vi "Boiler.vi"() -> ()   [LabVIEW 2013]
doc: "This VI is a simulation of boiler controller.\nThere are the following states-\n-Initialize\n-Reset Lockout\n-Pre-purge\n-Pre-purge continued\n-Ignition\n-Prove the pilot\n-Start and Run\n-Start and Run contiuued\n-Shutdown and purge: After elapsed time of the state VI will again go back to the initialize state.\n-Stop: On pressing Stop the VI will stop working and all the controlls and indicator will go to default value.\n\nThis VI allow the user to start and stop the boiller.\nThe status is a event string.\nTime Count- count the time till the time elapsed."
uses:
  Controls/Boiler Controls.ctl
  Controls/Boiler Simulation Controls.ctl
  Controls/Boiler Status Indicators.ctl
  CarWash/USB Template (LV 8.6)/Car Wash/Controls/States.ctl
panel:
  in  "Stop":bool
  out "Boiler Status Indicators":T1 {"Time Count" format="%.2g"}
  in  "Boiler Simulation Controls":T2 {"Flame Sensor Value (%)" min=0.0 max=100.0 scale=0.0..100.0}
  in  "Boiler Controls":T3 {"Fuel Valve Position" min=0.0 max=100.0 scale=0.0..100.0 scale format="%.2f"}
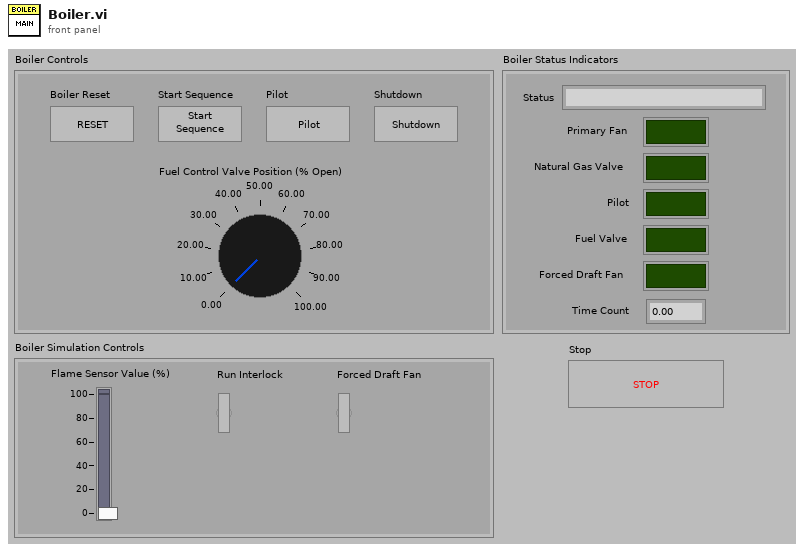
[diagram p1: front panel]
types:
  T1 = typedef "Boiler Status Indicators.ctl" = cluster{"Status":string, "Primary Fan":bool, "Natural Gas Valve":bool, "Pilot":bool, "Fuel Valve":bool, "Forced Draft Fan":bool, "Time Count":dbl}
  T2 = typedef "Boiler Simulation Controls.ctl" = cluster{"Flame Sensor Value (%)":dbl, "Run Interlock":bool, "Forced Draft Fan":bool}
  T3 = typedef "Boiler Controls.ctl" = cluster{"Boiler Reset":bool, "Start Sequence":bool, "Pilot":bool, "Shutdown":bool, "Fuel Valve Position":dbl}
  T4 = typedef "States.ctl" = enum16{"Initialize", "Start", "Reset Lockout", "Pre-Purge", "Pre-Perge Cont.", "Ignition", "Prove the Pilot", "Start and Run", "Run Cont.", "Shutdown and purge", "Purge", "Stop"}
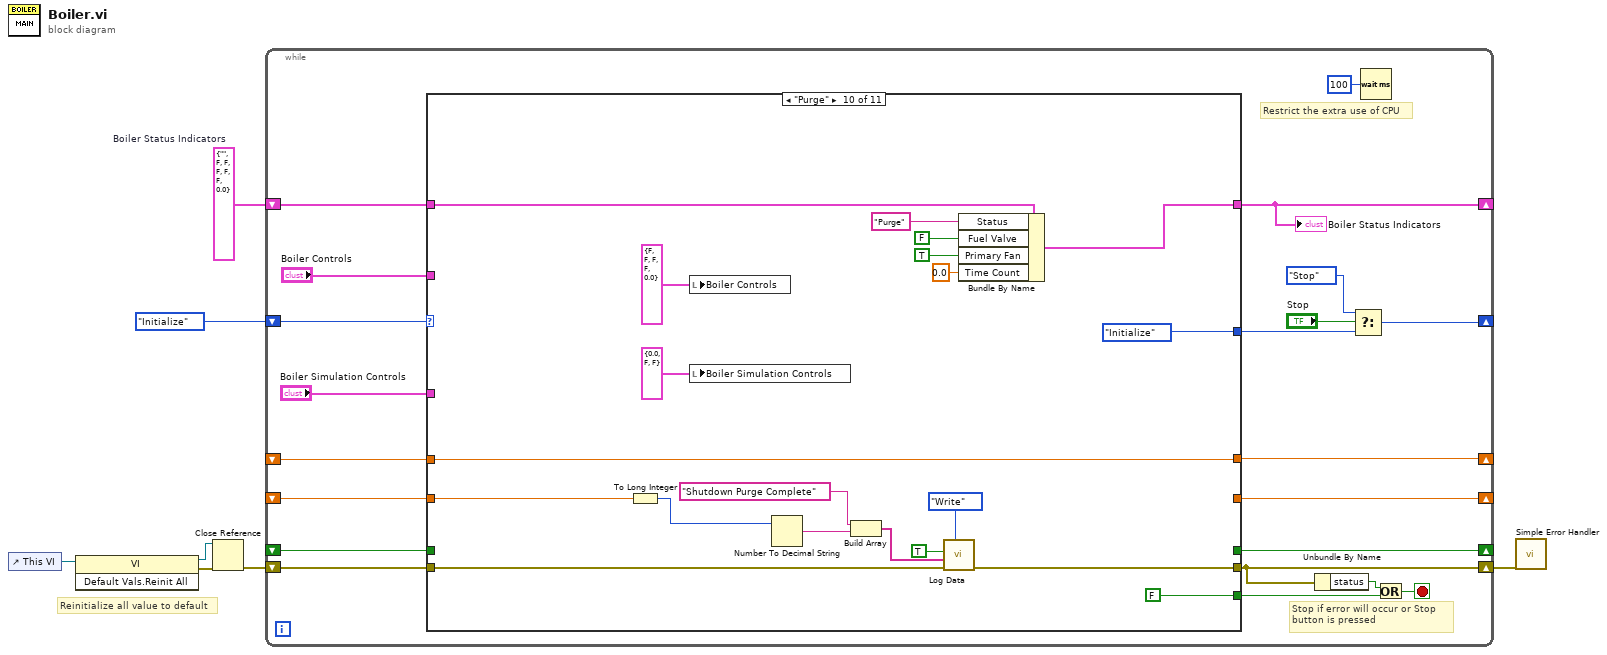
[diagram p0: block diagram]
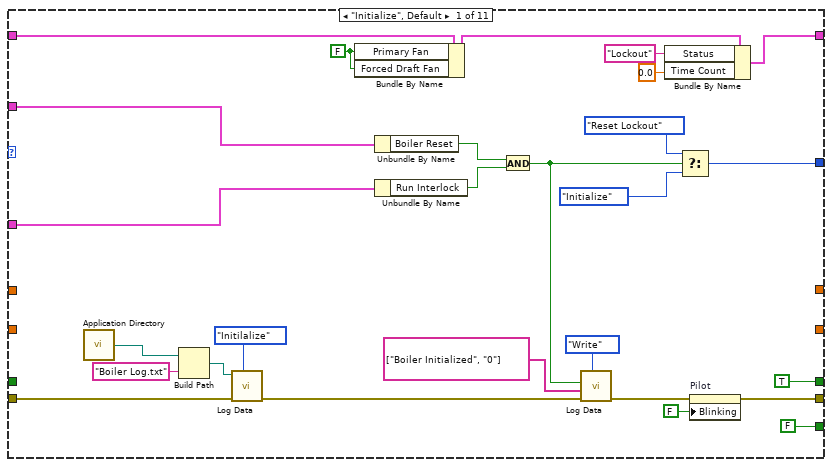
[diagram p2: hidden frame]
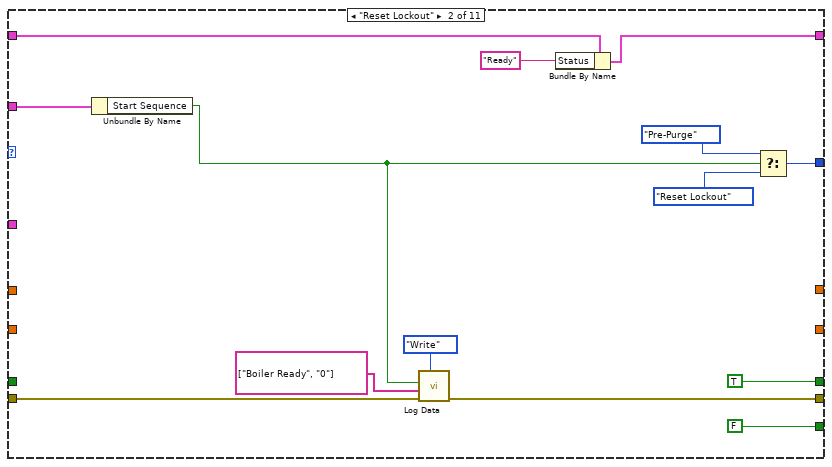
[diagram p3: hidden frame]
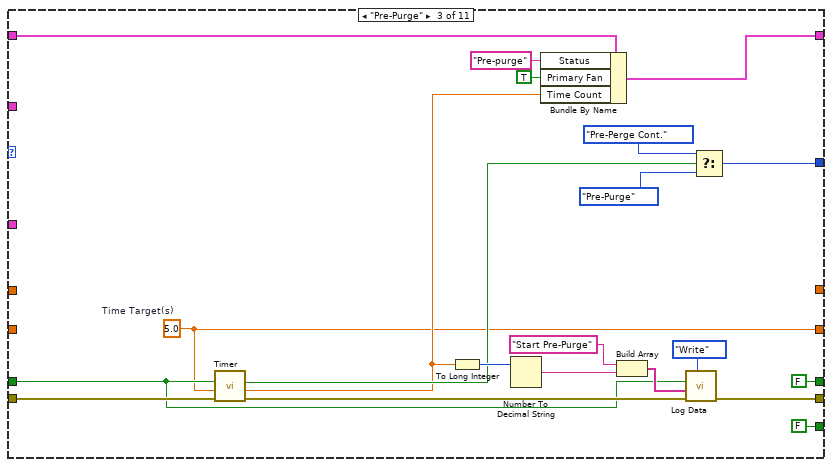
[diagram p4: hidden frame]
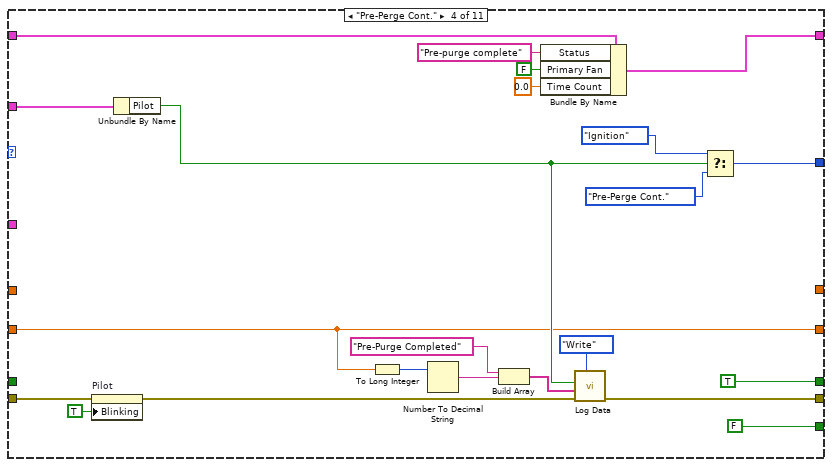
[diagram p5: hidden frame]
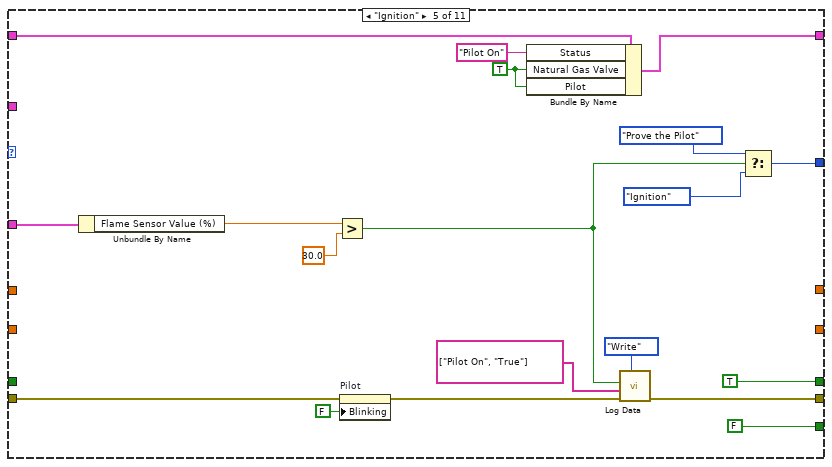
[diagram p6: hidden frame]
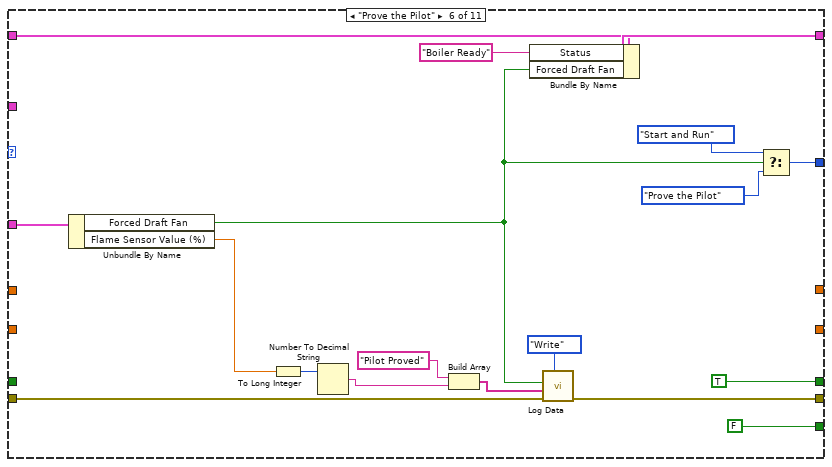
[diagram p7: hidden frame]
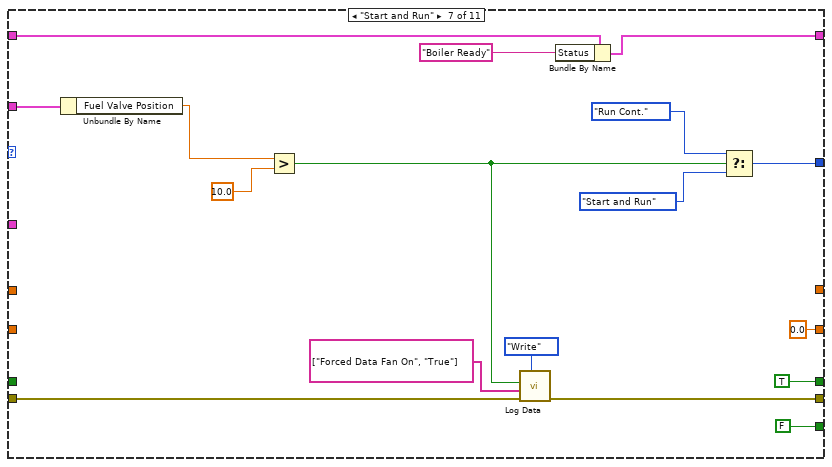
[diagram p8: hidden frame]
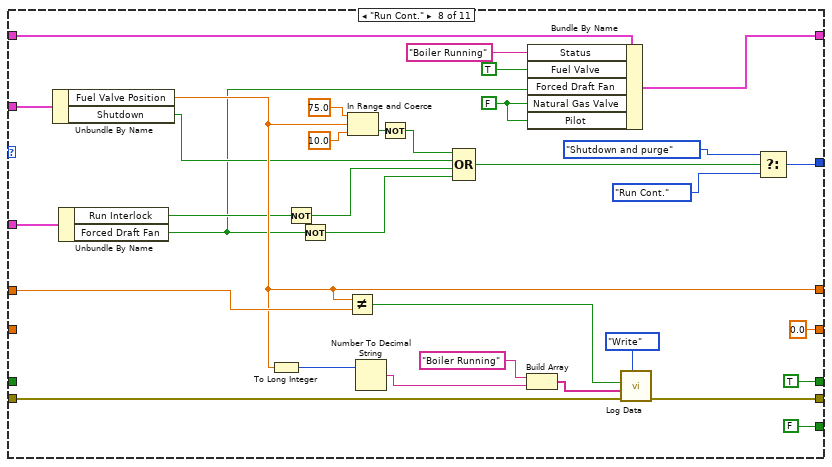
[diagram p9: hidden frame]
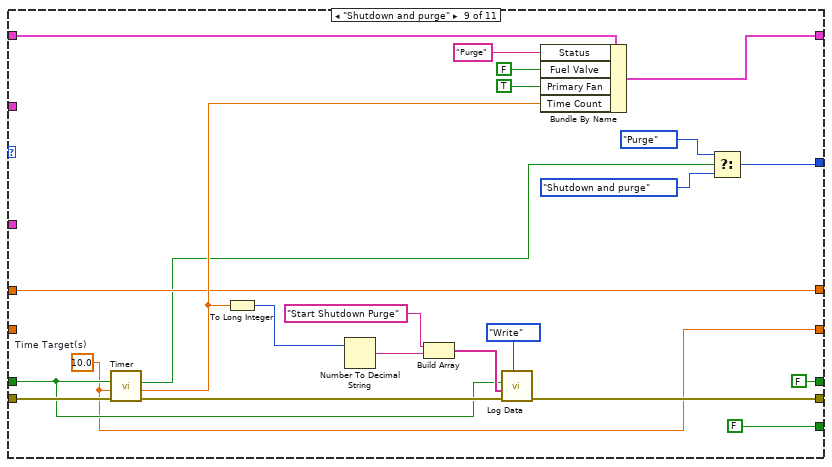
[diagram p10: hidden frame]
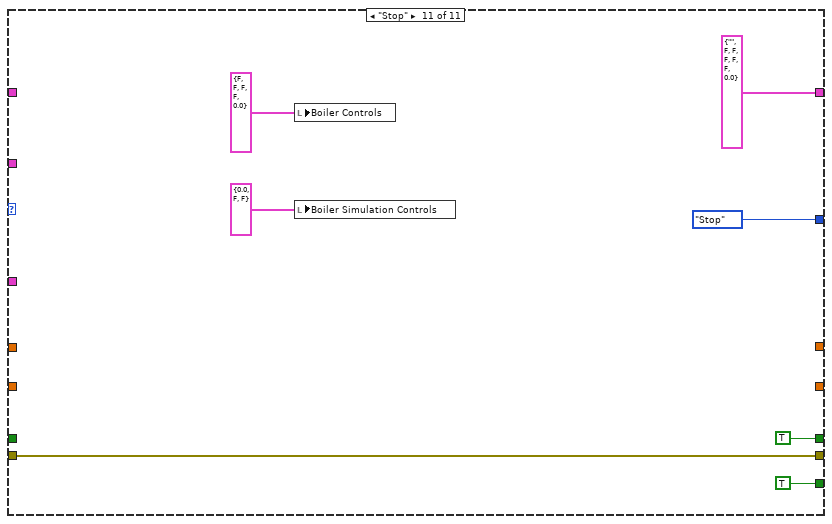
[diagram p11: hidden frame]
diagram:
  w2 = T1 {"Status"="", "Primary Fan"=FALSE, "Natural Gas Valve"=FALSE, "Pilot"=FALSE, "Fuel Valve"=FALSE, "Forced Draft Fan"=FALSE, "Time Count"=0.0}  # Boiler Status Indicators
  # "Reinitialize all value to default"
  n1 = control-ref of="This VI"() -> (w7:refnum<vi>)
  n2 = invoke class="VI" method="Default Vals.Reinit All"(reference=w7) -> (reference out=w5:refnum<vi>, error out=w6:errorcluster)  [unwired: 2 in, 1 out]
  n3 = Close Reference(reference=w5, error in (no error)=w6) -> (error out=w4:errorcluster)
  n4 = while {
    shift-right: [w27] -> w1
    shift-left: w4 -> [w28]
    shift-right: [w13] -> _
    shift-left: States."Initialize" -> [w23]
    shift-right: [w21] -> _
    shift-left: w2 -> [w22]
    shift-right: [w17] -> _
    shift-left: _ -> [w16]
    shift-right: [w11] -> _
    shift-left: _ -> [w10]
    shift-right: [w9] -> _
    shift-left: _ -> [w8]
    stop <- w26 stop-if-true
    # "Restrict the extra use of CPU"
    # "Stop if error will occur or Stop \nbutton is pressed"
    n5 = case shown="\"Purge\"" w23 {
      tunnel: [w45 w60 w80 w99 w119 w141 w157 w188 w213 w235 w245] -> w27
      tunnel: w28 -> [w43 w61 w83 w104 w126 w142 w158 w190 w217 w237 w245]
      tunnel: [FALSE FALSE FALSE FALSE FALSE FALSE FALSE FALSE FALSE FALSE TRUE] -> w24
      tunnel: [w53 w69 w90 w112 w131 w149 w166 w199 w222 w242 T1 {"Status"="", "Primary Fan"=FALSE, "Natural Gas Valve"=FALSE, "Pilot"=FALSE, "Fuel Valve"=FALSE, "Forced Draft Fan"=FALSE, "Time Count"=0.0} ("Boiler Status Indicators")] -> w21
      tunnel: w22 -> [w54 w68 w89 w111 w130 w148 w165 w198 w221 w241 _]
      tunnel: "Boiler Simulation Controls" -> [w51 _ _ _ w123 w144 _ w191 _ _ _]
      tunnel: [w48 w64 w86 w94 w115 w135 w155 w170 w206 States."Initialize" States."Stop"] -> w15
      tunnel: "Boiler Controls" -> [w34 w57 _ w102 _ _ w161 w192 _ _ _]
      tunnel: [TRUE TRUE ("Elapsed?") FALSE ("Elapsed?") TRUE ("Elapsed?") TRUE ("Elapsed?") TRUE ("Elapsed?") TRUE ("Elapsed?") TRUE ("Elapsed?") FALSE ("Elapsed?") _ TRUE ("Elapsed?")] -> w17
      tunnel: w16 -> [_ _ w73 _ _ _ _ _ w202 _ _]
      tunnel: [_ _ w70 w91 _ _ 0.0 ("Time Target(s)") 0.0 ("Time Target(s)") w201 _ _] -> w11
      tunnel: w10 -> [_ _ _ w91 _ _ _ _ _ w227 _]
      tunnel: [_ _ _ _ _ _ _ w180 w209 w234 _] -> w9
      tunnel: w8 -> [_ _ _ _ _ _ _ w182 w209 w234 _]
      frame "Initialize", Default {
        w29 = FALSE ("Primary Fan")
        n6 = call <vilib>:"Application Directory.vi"() -> ("Application Directory"=w42:path)
        n7 = Build Path(base path=w42, name or relative path="Boiler Log.txt") -> (appended path=w40:path)
        n8 = call "Log Data.vi"("Command"=enum16{"Initilalize", "Write", "Close"}."Initilalize", "error in (no error)"=w43, "file path"=w40) -> ("error out"=w38:errorcluster)  [unwired: 8 in]
        n9 = Bundle By Name(cluster=w54, "Primary Fan"=w29, "Forced Draft Fan"=w29) -> (w30:T1)
        n10 = Unbundle By Name(w34) -> ("Boiler Reset"=w33:bool)
        n11 = Unbundle By Name(w51) -> ("Run Interlock"=w32:bool)
        n12 = And(x=w33, y=w32) -> (x .and. y?=w31:bool)
        n13 = call "Log Data.vi"("Command"=enum16{"Initilalize", "Write", "Close"}."Write", "error in (no error)"=w38, "Array"=string[] ["Boiler Initialized", "0"], "Boolean"=w31) -> ("error out"=w37:errorcluster)  [unwired: 7 in]
        n14 = Bundle By Name(cluster=w30, "Status"="Lockout", "Time Count"=0.0) -> (w53:T1)
        n15 = Select(t=States."Reset Lockout", s=w31, f=States."Initialize") -> (s? t:f=w48:T4)
        n16 = property on="Pilot" class="Bool (strict)"(error in=w37, "Blinking"=FALSE) -> (error out=w45:errorcluster)  [unwired: 1 in, 1 out]
      }
      frame "Reset Lockout" {
        n17 = Unbundle By Name(w57) -> ("Start Sequence"=w56:bool)
        n18 = call "Log Data.vi"("Command"=enum16{"Initilalize", "Write", "Close"}."Write", "error in (no error)"=w61, "Array"=string[] ["Boiler Ready", "0"], "Boolean"=w56) -> ("error out"=w60:errorcluster)  [unwired: 7 in]
        n19 = Bundle By Name(cluster=w68, "Status"="Ready") -> (w69:T1)
        n20 = Select(t=States."Pre-Purge", s=w56, f=States."Reset Lockout") -> (s? t:f=w64:T4)
      }
      frame "Pre-Purge" {
        w70 = 5.0  # Time Target(s)
        n21 = call "Timer.vi"("error in (no error)"=w83, "Time Target(s)"=w70, "Reset"=w73) -> ("error out"=w81:errorcluster, "Elapsed TIme"=w71:dbl, "Elapsed?"=w74:bool)  [unwired: 6 in]
        n22 = To Long Integer(number=w71) -> (32bit integer=w79:i32)
        n23 = Number To Decimal String(number=w79) -> (decimal integer string=w78:string)  [unwired: 1 in]
        n24 = Bundle By Name(cluster=w89, "Status"="Pre-purge", "Primary Fan"=TRUE, "Time Count"=w71) -> (w90:T1)
        n25 = Build Array("Start Pre-Purge", w78) -> (w76:string[])
        n26 = call "Log Data.vi"("Command"=enum16{"Initilalize", "Write", "Close"}."Write", "error in (no error)"=w81, "Array"=w76, "Boolean"=w73) -> ("error out"=w80:errorcluster)  [unwired: 7 in]
        n27 = Select(t=States."Pre-Perge Cont.", s=w74, f=States."Pre-Purge") -> (s? t:f=w86:T4)
      }
      frame "Pre-Perge Cont." {
        n28 = property on="Pilot" class="Bool (strict)"(error in=w104, "Blinking"=TRUE) -> (error out=w100:errorcluster)  [unwired: 1 in, 1 out]
        n29 = Unbundle By Name(w102) -> ("Pilot"=w92:bool)
        n30 = To Long Integer(number=w91) -> (32bit integer=w98:i32)
        n31 = Number To Decimal String(number=w98) -> (decimal integer string=w97:string)  [unwired: 1 in]
        n32 = Build Array("Pre-Purge Completed", w97) -> (w96:string[])
        n33 = Bundle By Name(cluster=w111, "Status"="Pre-purge complete", "Primary Fan"=FALSE, "Time Count"=0.0) -> (w112:T1)
        n34 = call "Log Data.vi"("Command"=enum16{"Initilalize", "Write", "Close"}."Write", "error in (no error)"=w100, "Array"=w96, "Boolean"=w92) -> ("error out"=w99:errorcluster)  [unwired: 7 in]
        n35 = Select(t=States."Ignition", s=w92, f=States."Pre-Perge Cont.") -> (s? t:f=w94:T4)
      }
      frame "Ignition" {
        w124 = TRUE ("Primary Fan")
        n36 = Unbundle By Name(w123) -> ("Flame Sensor Value (%)"=w122:dbl)
        n37 = Greater?(x=w122, y=30.0) -> (0:w114:bool)
        n38 = property on="Pilot" class="Bool (strict)"(error in=w126, "Blinking"=FALSE) -> (error out=w120:errorcluster)  [unwired: 1 in, 1 out]
        n39 = Bundle By Name(cluster=w130, "Status"="Pilot On", "Natural Gas Valve"=w124, "Pilot"=w124) -> (w131:T1)
        n40 = call "Log Data.vi"("Command"=enum16{"Initilalize", "Write", "Close"}."Write", "error in (no error)"=w120, "Array"=string[] ["Pilot On", "True"], "Boolean"=w114) -> ("error out"=w119:errorcluster)  [unwired: 7 in]
        n41 = Select(t=States."Prove the Pilot", s=w114, f=States."Ignition") -> (s? t:f=w115:T4)
      }
      frame "Prove the Pilot" {
        n42 = Unbundle By Name(w144) -> ("Forced Draft Fan"=w132:bool, "Flame Sensor Value (%)"=w139:dbl)
        n43 = To Long Integer(number=w139) -> (32bit integer=w138:i32)
        n44 = Number To Decimal String(number=w138) -> (decimal integer string=w140:string)  [unwired: 1 in]
        n45 = Build Array("Pilot Proved", w140) -> (w134:string[])
        n46 = Bundle By Name(cluster=w148, "Status"="Boiler Ready", "Forced Draft Fan"=w132) -> (w149:T1)
        n47 = call "Log Data.vi"("Command"=enum16{"Initilalize", "Write", "Close"}."Write", "error in (no error)"=w142, "Array"=w134, "Boolean"=w132) -> ("error out"=w141:errorcluster)  [unwired: 7 in]
        n48 = Select(t=States."Start and Run", s=w132, f=States."Prove the Pilot") -> (s? t:f=w135:T4)
      }
      frame "Start and Run" {
        n49 = Unbundle By Name(w161) -> ("Fuel Valve Position"=w160:dbl)
        n50 = Greater?(x=w160, y=10.0) -> (0:w152:bool)
        n51 = call "Log Data.vi"("Command"=enum16{"Initilalize", "Write", "Close"}."Write", "error in (no error)"=w158, "Array"=string[] ["Forced Data Fan On", "True"], "Boolean"=w152) -> ("error out"=w157:errorcluster)  [unwired: 7 in]
        n52 = Bundle By Name(cluster=w165, "Status"="Boiler Ready") -> (w166:T1)
        n53 = Select(t=States."Run Cont.", s=w152, f=States."Start and Run") -> (s? t:f=w155:T4)
      }
      frame "Run Cont." {
        w193 = FALSE ("Forced Draft Fan")
        n54 = Unbundle By Name(w192) -> ("Fuel Valve Position"=w180:dbl, "Shutdown"=w176:bool)
        n55 = Unbundle By Name(w191) -> ("Run Interlock"=w175:bool, "Forced Draft Fan"=w169:bool)
        n56 = To Long Integer(number=w180) -> (32bit integer=w186:i32)
        n57 = Not(x=w175) -> (.not. x?=w174:bool)
        n58 = Not(x=w169) -> (.not. x?=w173:bool)
        n59 = Not Equal?(x=w180, y=w182) -> (x != y?=w181:bool)
        n60 = In Range and Coerce(upper limit=75.0, x=w180, lower limit=10.0) -> (In Range?=w177:bool)  [unwired: 1 out]
        n61 = Number To Decimal String(number=w186) -> (decimal integer string=w187:string)  [unwired: 1 in]
        n62 = Not(x=w177) -> (.not. x?=w167:bool)
        n63 = Compound Arithmetic op=OR(w167, w176, w174, w173) -> (w168:bool)
        n64 = Build Array("Boiler Running", w187) -> (w183:string[])
        n65 = Bundle By Name(cluster=w198, "Status"="Boiler Running", "Fuel Valve"=TRUE, "Forced Draft Fan"=w169, "Natural Gas Valve"=w193, "Pilot"=w193) -> (w199:T1)
        n66 = call "Log Data.vi"("Command"=enum16{"Initilalize", "Write", "Close"}."Write", "error in (no error)"=w190, "Array"=w183, "Boolean"=w181) -> ("error out"=w188:errorcluster)  [unwired: 7 in]
        n67 = Select(t=States."Shutdown and purge", s=w168, f=States."Run Cont.") -> (s? t:f=w170:T4)
      }
      frame "Shutdown and purge" {
        w201 = 10.0  # Time Target(s)
        n68 = call "Timer.vi"("error in (no error)"=w217, "Time Target(s)"=w201, "Reset"=w202) -> ("error out"=w215:errorcluster, "Elapsed TIme"=w211:dbl, "Elapsed?"=w203:bool)  [unwired: 6 in]
        n69 = To Long Integer(number=w211) -> (32bit integer=w210:i32)
        n70 = Number To Decimal String(number=w210) -> (decimal integer string=w212:string)  [unwired: 1 in]
        n71 = Build Array("Start Shutdown Purge", w212) -> (w208:string[])
        n72 = call "Log Data.vi"("Command"=enum16{"Initilalize", "Write", "Close"}."Write", "error in (no error)"=w215, "Array"=w208, "Boolean"=w202) -> ("error out"=w213:errorcluster)  [unwired: 7 in]
        n73 = Bundle By Name(cluster=w221, "Status"="Purge", "Fuel Valve"=FALSE, "Primary Fan"=TRUE, "Time Count"=w211) -> (w222:T1)
        n74 = Select(t=States."Purge", s=w203, f=States."Shutdown and purge") -> (s? t:f=w206:T4)
      }
      frame "Purge" {
        n75 = To Long Integer(number=w227) -> (32bit integer=w228:i32)
        n76 = local write "Boiler Controls"(T3 {"Boiler Reset"=FALSE, "Start Sequence"=FALSE, "Pilot"=FALSE, "Shutdown"=FALSE, "Fuel Valve Position"=0.0} ("Boiler Controls")) -> ()
        n77 = local write "Boiler Simulation Controls"(T2 {"Flame Sensor Value (%)"=0.0, "Run Interlock"=FALSE, "Forced Draft Fan"=FALSE} ("Boiler Simulation Controls")) -> ()
        n78 = Number To Decimal String(number=w228) -> (decimal integer string=w229:string)  [unwired: 1 in]
        n79 = Build Array("Shutdown Purge Complete", w229) -> (w226:string[])
        n80 = call "Log Data.vi"("Command"=enum16{"Initilalize", "Write", "Close"}."Write", "error in (no error)"=w237, "Array"=w226, "Boolean"=TRUE) -> ("error out"=w235:errorcluster)  [unwired: 7 in]
        n81 = Bundle By Name(cluster=w241, "Status"="Purge", "Fuel Valve"=FALSE, "Primary Fan"=TRUE, "Time Count"=0.0) -> (w242:T1)
      }
      frame "Stop" {
        n82 = local write "Boiler Controls"(T3 {"Boiler Reset"=FALSE, "Start Sequence"=FALSE, "Pilot"=FALSE, "Shutdown"=FALSE, "Fuel Valve Position"=0.0} ("Boiler Controls")) -> ()
        n83 = local write "Boiler Simulation Controls"(T2 {"Flame Sensor Value (%)"=0.0, "Run Interlock"=FALSE, "Forced Draft Fan"=FALSE} ("Boiler Simulation Controls")) -> ()
      }
    }
    "Boiler Status Indicators" <- w21
    n84 = Unbundle By Name(w27) -> ("status"=w25:bool)
    n85 = Select(t=States."Stop", s="Stop", f=w15) -> (s? t:f=w13:T4)
    n86 = Wait (ms)(milliseconds to wait=u32 100) -> ()  [unwired: 1 out]
    n87 = Or(x=w25, y=w24) -> (x .or. y?=w26:bool)
  }
  n88 = call <vilib>:"Simple Error Handler.vi"("error in (no error)"=w1) -> ()  [unwired: 4 in, 5 out]
